vi "close.vi"(8 "error in (no error)":errorcluster, 11 "DS360 in":refnum<class "DS360.lvclass">) -> (0 "error out":errorcluster, 3 "DS360 out":refnum<class "DS360.lvclass">)   [LabVIEW 2019, in "DS360.lvclass"]
uses:
  DS360.lvclass
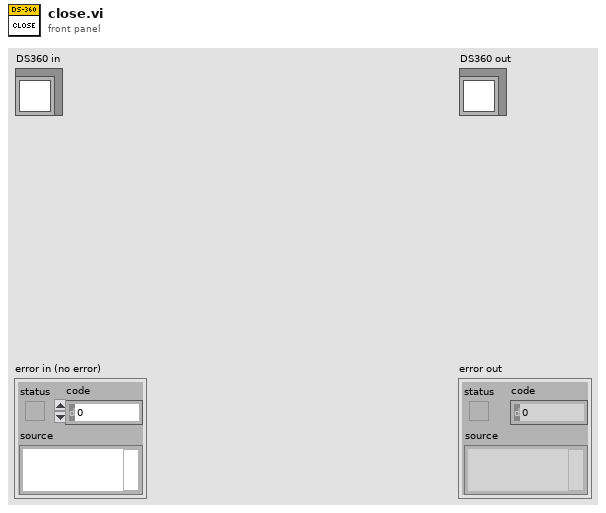
[diagram p1: front panel]
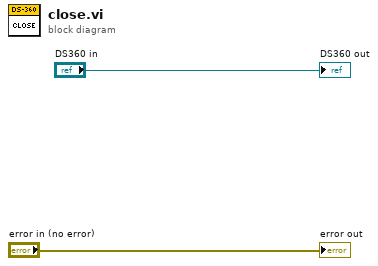
[diagram p0: block diagram]
diagram:
  "error out" <- "error in (no error)"
  "DS360 out" <- "DS360 in"
